vi "Write Files.vi"(8 "error in (no error)":errorcluster, 10 "Files":path[](array[path]), 11 "XY WFRM Plot in":refnum<class "XY WFRM Plot.lvclass">) -> (0 "error out":errorcluster, 3 "XY WFRM Plot out":refnum<class "XY WFRM Plot.lvclass">)   [LabVIEW 2018, in "XY WFRM Plot.lvclass"]
uses:
  XY WFRM Plot.lvclass
  C:/github/LabActor/Plots/Plot/Plot.lvclass
  Plot/Plot.lvclass/Plot.ctl
  XY WFRM Plot.lvclass/XY WFRM Plot.ctl
  Read Files ref.vi
  Plot/Read Files.vi
  Plot/Plot.lvclass
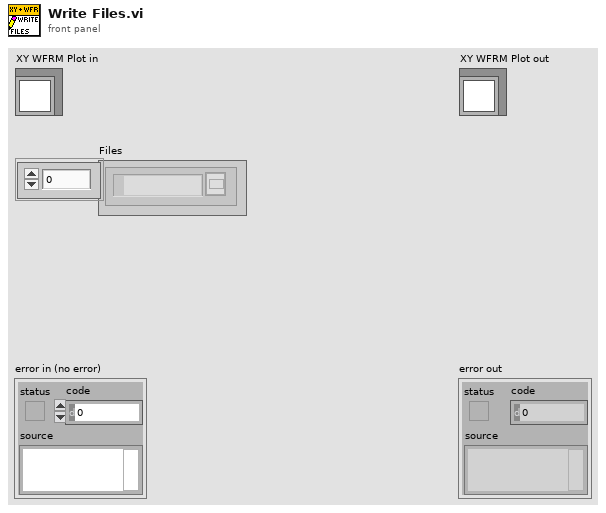
[diagram p1: front panel]
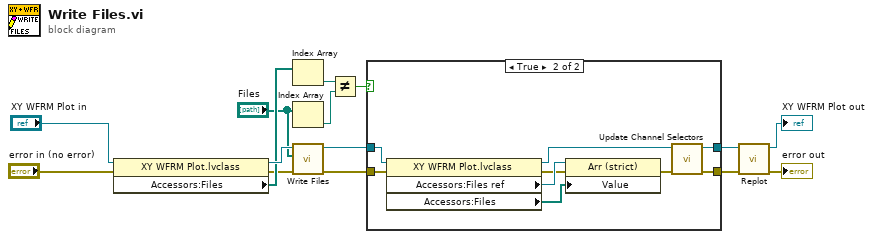
[diagram p0: block diagram]
diagram:
  n1 = property class="XY WFRM Plot.lvclass"(reference="XY WFRM Plot in", error in="error in (no error)") -> (reference out=w14:refnum<class "XY WFRM Plot.lvclass">, error out=w5:errorcluster, "Accessors:Files"=w13:path[])
  n2 = Index Array(array=w13) -> (element=w11:path)  [unwired: 1 in]
  n3 = Index Array(array="Files") -> (element=w10:path)  [unwired: 1 in]
  n4 = call-parent "Write Files.vi"("error in (no error)"=w5, "Files"="Files", "Plot in"=w14) -> ("error out"=w8:errorcluster, "Plot out"=w9:refnum<class "XY WFRM Plot.lvclass">)  [unwired: 7 in]
  n5 = Not Equal?(x=w11, y=w10) -> (x != y?=w7:bool)
  n6 = case shown="True" w7 {
    tunnel: w9 -> [w17 w26]
    tunnel: [w17 w20] -> w6
    tunnel: w8 -> [w16 w24]
    tunnel: [w16 w18] -> w2
    frame False {
    }
    frame True {
      n7 = property class="XY WFRM Plot.lvclass"(reference=w26, error in=w24) -> (reference out=w25:refnum<class "XY WFRM Plot.lvclass">, error out=w22:errorcluster, "Accessors:Files ref"=w23:refnum<vi>, "Accessors:Files"=w21:path[])
      n8 = property class="Arr (strict)"(reference=w23, error in=w22, "Value"=w21) -> (error out=w19:errorcluster)  [unwired: 1 out]
      n9 = call-dynamic "Update Channel Selectors.vi"("error in (no error)"=w19, "XY WFRM Plot in"=w25) -> ("error out"=w18:errorcluster, "XY WFRM Plot out"=w20:refnum<class "XY WFRM Plot.lvclass">)  [unwired: 8 in]
    }
  }
  n10 = call-dynamic "Replot.vi"("error in (no error)"=w2, "Plot in"=w6) -> ("error out"=→"error out":errorcluster, "Plot out"=→"XY WFRM Plot out":refnum<class "XY WFRM Plot.lvclass">)  [unwired: 8 in]
